vi "ILAB_CaseHandler.vi"(4 "data":string, 5 "action":string) -> (0 "errorOut":string, 1 "response":string)   [LabVIEW 2009]
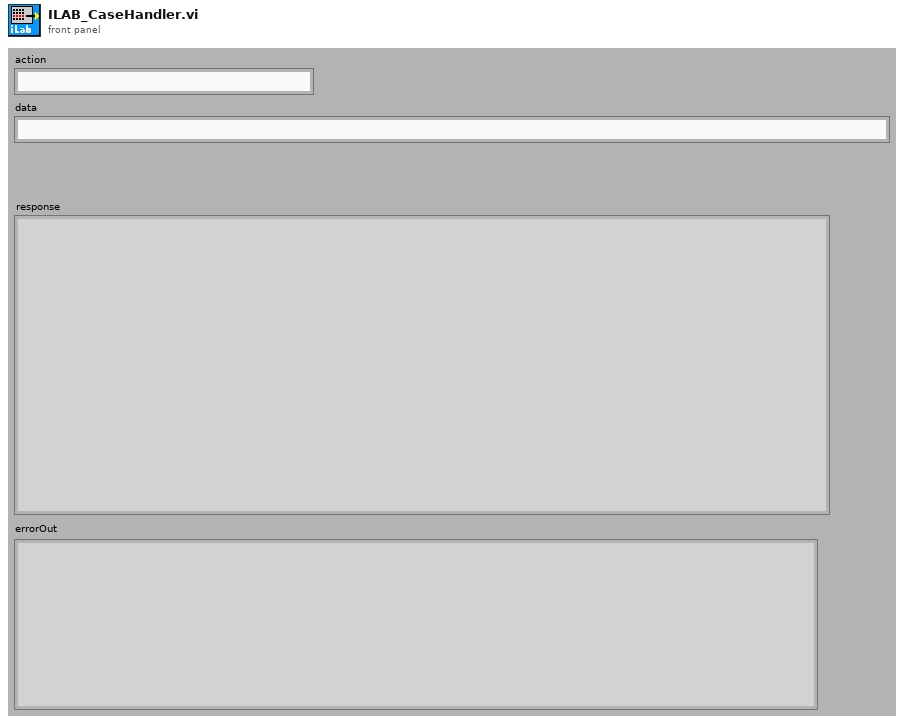
[diagram p1: front panel]
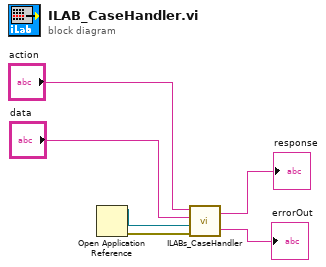
[diagram p0: block diagram]
diagram:
  n1 = Open Application Reference() -> (0:w4:errorcluster, 3:w3:refnum<vi>)  [unwired: 1 in, 3 out]
  n2 = call "ILABs_CaseHandler.vi"("error In"=w4, "appReference"=w3, "data"="data", "action"="action") -> ("errorOut"=→"errorOut":string, "response"=→"response":string)
